vi "setUp.vi"(8 "error in (no error)":errorcluster, 11 "reference in":refnum<class "Add and Remove Test.lvclass">) -> (0 "error out":errorcluster, 3 "reference out":refnum<class "Add and Remove Test.lvclass">)   [LabVIEW 2017, in "Add and Remove Test.lvclass"]
doc: "setUp runs prior to the test method during test execution. Use this method to initialize any object data required by your tests."
uses:
  Add and Remove Test.lvclass
  C:/Program Files (x86)/National Instruments/LabVIEW 2017/vi.lib/addons/_JKI Toolkits/VI Tester/TestCase.llb/TestCase.lvclass
  NationalInstruments.VeriStand.SystemDefinitionAPI
  Add and Remove Test.lvclass/Add and Remove Test.ctl
  <vilib>/addons/_JKI Toolkits/VI Tester/TestCase.llb/TestCase.lvclass
  niveristand-custom-device-testing-tools/VeriStandTestUtilities/VeriStandTestUtilities.lvlib
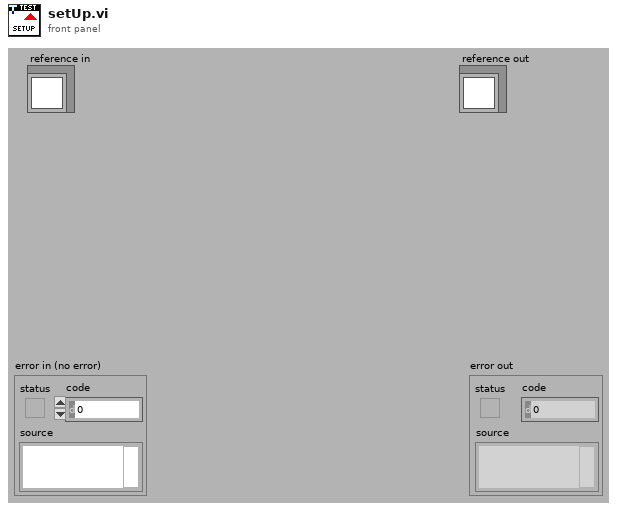
[diagram p1: front panel]
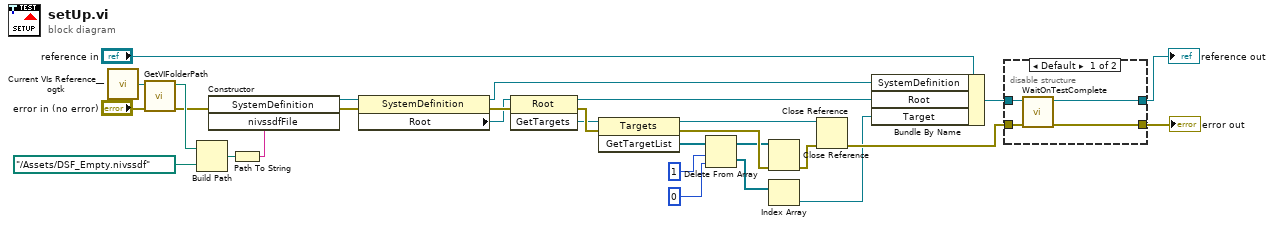
[diagram p0: block diagram]
diagram:
  n1 = call <userlib>:"Current VIs Reference__ogtk.vi"() -> ("Current VI's reference"=w29:refnum<vi>)  [unwired: 5 in]
  n2 = call "GetVIFolderPath.vi"("error in (no error)"="error in (no error)", "VI Reference in"=w29) -> ("error out"=w25:errorcluster, "VI Folder Path out"=w28:path)  [unwired: 8 in]
  n3 = Build Path(base path=w28, name or relative path=path "../Assets/DSF_Empty.nivssdf" ("Absolute or Relative Path")) -> (appended path=w26:path)
  n4 = Path To String(path=w26) -> (string=w23:string)
  n5 = constructor class="SystemDefinition" ("Constructor Node")(error in=w25, "nivssdfFile"=w23) -> (reference out=w22:refnum<k24>, error out=w24:errorcluster)  [unwired: 2 in, 2 out]
  n6 = property on="Property Node" class="SystemDefinition"(reference=w22, error in=w24) -> (reference out=w3:refnum<k24>, error out=w21:errorcluster, "Root"=w20:refnum<k24>)
  n7 = invoke on="Invoke Node" class="Root" method="GetTargets"(reference=w20, error in=w21) -> (reference out=w2:refnum<k24>, error out=w19:errorcluster, "GetTargets"=w18:refnum<k24>)  [unwired: 1 in]
  n8 = invoke on="Invoke Node" class="Targets" method="GetTargetList"(reference=w18, error in=w19) -> (reference out=w11:refnum<k24>, error out=w14:errorcluster, "GetTargetList"=w17:refnum<k24>[])  [unwired: 1 in]
  n9 = Delete From Array(array=w17, length=1, index=0) -> (deleted portion=w10:refnum<k24>[], array with subset deleted=w13:refnum<k24>[])
  n10 = Close Reference(reference=w13, error in (no error)=w14) -> (error out=w12:errorcluster)
  n11 = Index Array(array=w10) -> (element=w1:refnum<k24>)  [unwired: 1 in]
  n12 = Close Reference(reference=w11, error in (no error)=w12) -> (error out=w8:errorcluster)
  n13 = Bundle By Name(cluster="reference in", "SystemDefinition"=w3, "Root"=w2, "Target"=w1) -> (w9:refnum<class "Add and Remove Test.lvclass">)
  n14 = disable-structure "Conditional Disable Structure" shown="Default" {
    disable-tunnel: w8 -> [w33 w34]
    disable-tunnel: [w32 w34] -> w5
    disable-tunnel: [w31 w35] -> w4
    disable-tunnel: w9 -> [w30 w35]
    frame condition #0 (active) {
      n15 = call <vilib>:"WaitOnTestComplete.vi"("error in (no error)"=w33, "TestCase in"=w30) -> ("error out"=w32:errorcluster, "TestCase out"=w31:refnum<class "Add and Remove Test.lvclass">)  [unwired: 8 in]
    }
    frame condition #1 {
    }
  }
  "error out" <- w5
  "reference out" <- w4
